vi "Control Experiment FGV.vi"(6 "Function":enum16{"read", "write"}(ring), 8 "error in (no error)":errorcluster, 10 "Cluster in":T1) -> (0 "error out":errorcluster, 2 "Cluster out":T1)   [LabVIEW 2016, in "Transport.lvclass"]
uses:
  Transport.lvclass
  Control Experiment FGV-cluster.ctl
  <userlib>/LevyLab/Krohn Hite 7008/typedefs/Gain-Enum.ctl
  <userlib>/LevyLab/Krohn Hite 7008/typedefs/Shunt-Enum.ctl
  <userlib>/LevyLab/Krohn Hite 7008/KH7008.lvclass
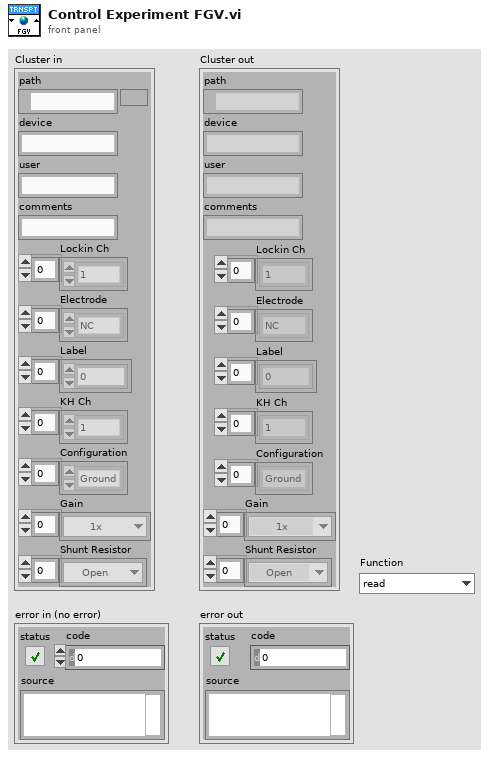
[diagram p1: front panel]
types:
  T1 = typedef "Control Experiment FGV-cluster.ctl" = cluster{"path":path, "device":string, "user":string, "comments":string, "Lockin Ch":enum16{"1", "2", "3", "4", "5", "6", "7", "8"}[], "Electrode":enum16{"NC", "26", "27", "28", "1", "2", "3", "4", "5", "6", "7", "8", "9", "10", "11", "12", "13", "14", "15", "16", "17", "18", "19", "20", "21", "22", "23", "24", "25"}[], "Label":u16[], "KH Ch":enum16{"1", "2", "3", "4", "5", "6", "7", "8"}[], "Configuration":enum16{"Ground", "Current", "Voltage", "Gate"}[], "Gain":T2[], "Shunt Resistor":T3[]}
  T2 = typedef "KH7008.lvclass/Gain-Enum.ctl" = enum16{"1x", "10x", "100x", "1000x"}
  T3 = typedef "KH7008.lvclass/Shunt-Enum.ctl" = enum16{"Open", "50 Ohms", "500 Ohms", "5k Ohms", "50k Ohms"}
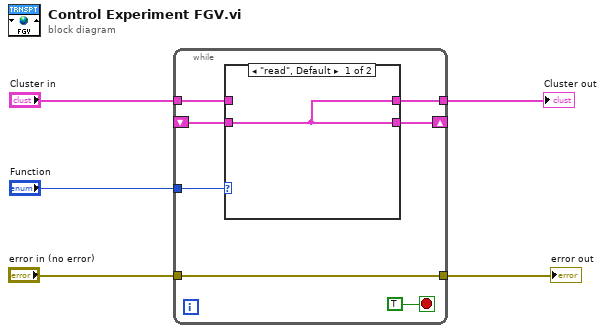
[diagram p0: block diagram]
diagram:
  n1 = while {
    tunnel: "Cluster in" -> [w8]
    tunnel: "error in (no error)" -> [w12]
    tunnel: [w12] -> w4
    tunnel: [w7] -> w5
    shift-right: [w9] -> _
    shift-left: _ -> [w6]
    tunnel: "Function" -> [w10]
    stop <- TRUE stop-if-true
    n2 = case shown="\"read\", Default" w10 {
      tunnel: [w13 w14] -> w9
      tunnel: w8 -> [_ w14]
      tunnel: [w13 w14] -> w7
      tunnel: w6 -> [w13 _]
      frame "read", Default {
      }
      frame "write" {
      }
    }
  }
  "Cluster out" <- w5
  "error out" <- w4
